vi "Countdown V1.4(SubVI).vi"(9 "start input":bool) -> (0 "timer out":dbl format="%<%M:%S>t")   [LabVIEW 2020]
panel:
  # "T"
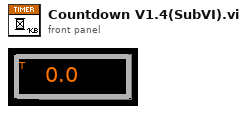
[diagram p1: front panel]
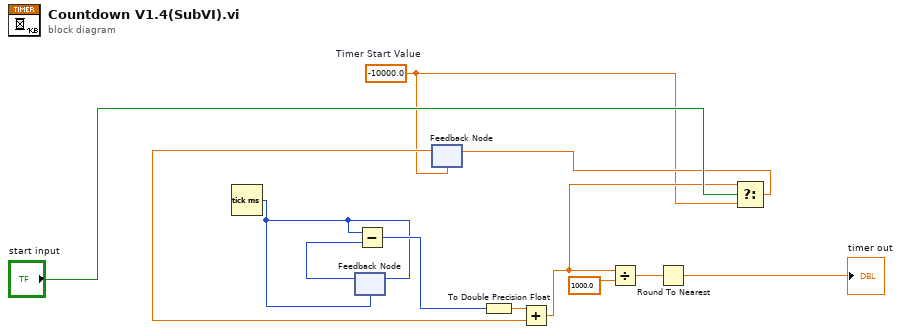
[diagram p0: block diagram]
diagram:
  w1 = -10000.0  # Timer Start Value
  n1 = Tick Count (ms)() -> (millisecond timer value=w2:u32)
  n2 = feedback #1(w2) -> (w4:u32)
  n3 = feedback-in #1(w2) -> ()
  n4 = Subtract(x=w2, y=w4) -> (x-y=w3:u32)
  n5 = feedback #2(w1) -> (w5:dbl)
  n6 = To Double Precision Float(number=w3) -> (double precision float=w10:dbl)
  n7 = Add(x=w10, y=w5) -> (x+y=w9:dbl)
  n8 = Divide(x=w9, y=1000.0) -> (x/y=w8:dbl)
  n9 = Round To Nearest(number=w8) -> (nearest integer value=→"timer out":dbl)
  n10 = Select(t=w9, s="start input", f=w1) -> (s? t:f=w6:dbl)
  n11 = feedback-in #2(w6) -> ()
